vi "Bottom segment value_test2.vi"(10 "Bottom player segment position":string) -> (1 "Bottom player segment":i32, 2 "Bottom player court segment display":bool[][](array[boolean]))   [LabVIEW 2013]
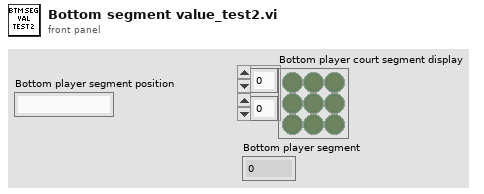
[diagram p1: front panel]
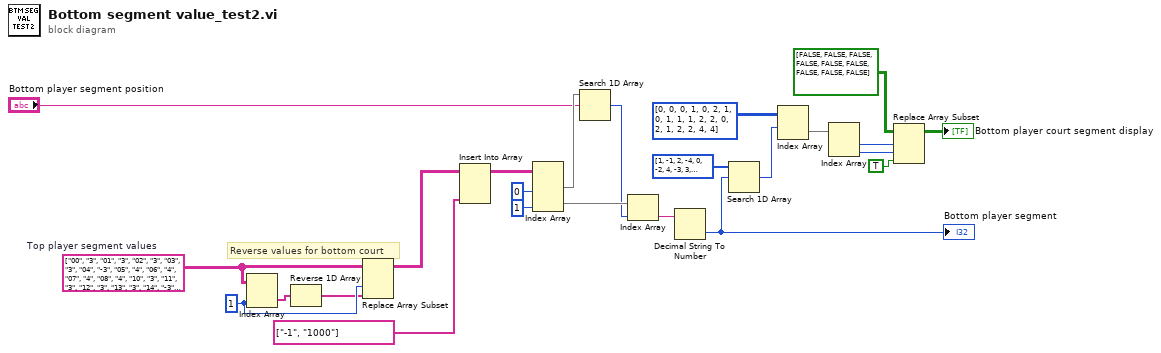
[diagram p0: block diagram]
diagram:
  w1 = string[][] [["00", "3"], ["01", "3"], ["02", "3"], ["03", "3"], ["04", "-3"], ["05", "4"], ["06", "4"], ["07", "4"], ["08", "4"], ["10", "3"], ["11", "3"], ["12", "3"], ["13", "3"], ["14", "-3"], ["15", "4"], ["16", "4"], ["17", "4"], ["18", "4"], ["20", "3"], ["21", "3"], ["22", "3"], ["23", "3"], ["24", "-3"], ["25", "4"], ["26", "4"], ["27", "4"], ["28", "4"], ["30", "3"], ["31", "3"], ["32", "3"], ["33", "0"], ["34", "0"], ["35", "0"], ["36", "4"], ["37", "4"], ["38", "4"], ["40", "-2"], ["41", "-2"], ["42", "-2"], ["43", "0"], ["44", "0"], ["45", "0"], ["46", "-4"], ["47", "-4"], ["48", "-4"], ["50", "2"], ["51", "2"], ["52", "2"], ["53", "0"], ["54", "0"], ["55", "0"], ["56", "1"], ["57", "1"], ["58", "1"], ["60", "2"], ["61", "2"], ["62", "2"], ["63", "2"], ["64", "-1"], ["65", "1"], ["66", "1"], ["67", "1"], ["68", "1"], ["70", "2"], ["71", "2"], ["72", "2"], ["73", "2"], ["74", "-1"], ["75", "1"], ["76", "1"], ["77", "1"], ["78", "1"], ["80", "2"], ["81", "2"], ["82", "2"], ["83", "2"], ["84", "-1"], ["85", "1"], ["86", "1"], ["87", "1"], ["88", "1"]]  # Top player segment values
  w16 = 1 ("disabled index (col)")
  # "Reverse values for bottom court"
  n1 = Index Array(array=w1, index (col)=w16) -> (element=w17:string[])  [unwired: 1 in]
  n2 = Reverse 1D Array(array=w17) -> (reversed array=w15:string[])
  n3 = Replace Array Subset(array=w1, new element=w15, index (col)=w16) -> (w13:string[][])  [unwired: 1 in]
  n4 = Insert Into Array(array=w13, new element=string[] ["-1", "1000"] ("new element/subarray")) -> (w12:string[][])  [unwired: 2 in]
  n5 = Index Array(array=w12, index (col) #1=0 ("disabled index (col)"), index (col) #2=1 ("index (col)")) -> (element #1=w23:string[], element #2=w20:string[])  [unwired: 2 in]
  n6 = Search 1D Array(1D array=w23, element="Bottom player segment position") -> (index of element=w19:i32)  [unwired: 1 in]
  n7 = Index Array(array=w20, index=w19) -> (element=w18:string)
  n8 = Decimal String To Number(string=w18) -> (number=w3:i32)  [unwired: 2 in, 1 out]
  "Bottom player segment" <- w3
  n9 = Search 1D Array(1D array=i32[] [1, -1, 2, -4, 0, -2, 4, -3, 3, 1000], element=w3) -> (index of element=w9:i32)  [unwired: 1 in]
  n10 = Index Array(array=i32[][] [[0, 0], [0, 1], [0, 2], [1, 0], [1, 1], [1, 2], [2, 0], [2, 1], [2, 2], [4, 4]], index (row)=w9) -> (element=w8:i32[])  [unwired: 1 in]
  n11 = Index Array(array=w8) -> (element #1=w6:i32, element #2=w5:i32)  [unwired: 2 in]
  n12 = Replace Array Subset(array=bool[][] [[FALSE, FALSE, FALSE], [FALSE, FALSE, FALSE], [FALSE, FALSE, FALSE]] ("Top player court segment display"), new element=TRUE ("new element/subarray"), index (row)=w6, index (col)=w5) -> (→"Bottom player court segment display":bool[][])
